vi "CameraScaleCoordToImgCoord.vi"(9 "value":dbl, 10 "img size":dbl, 11 "scale bounds":cluster{"min":i16, "max":i16}) -> (3 "coord out":i32)   [LabVIEW 2019]
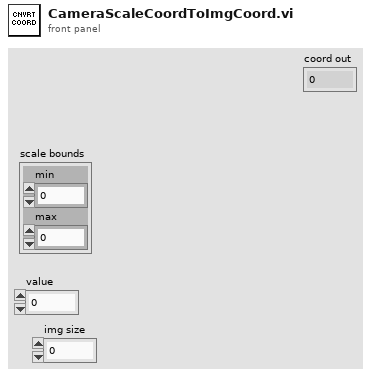
[diagram p1: front panel]
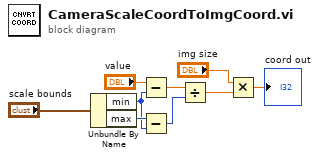
[diagram p0: block diagram]
diagram:
  n1 = Unbundle By Name("scale bounds") -> ("min"=w1:i16, "max"=w7:i16)
  n2 = Subtract(x="value", y=w1) -> (x-y=w8:dbl)
  n3 = Subtract(x=w7, y=w1) -> (x-y=w6:i16)
  n4 = Divide(x=w8, y=w6) -> (x/y=w5:dbl)
  n5 = Multiply(x="img size", y=w5) -> (x*y=→"coord out":dbl)
